vi "Intake_Execute.vi"() -> ()   [LabVIEW 2019]
uses:
  <vilib>/Rock Robotics/WPI/Solenoid/WPI_SolenoidValue.ctl
  Globals/Intake_Globals.vi
  <vilib>/Rock Robotics/WPI/ThirdParty/REV Robotics/SPARK MAX/Typedef/Spark MAX Control Type.ctl
panel:
  in  "Intake_Speed":dbl
  out "Intake_Extend":T1=enum."Reverse"
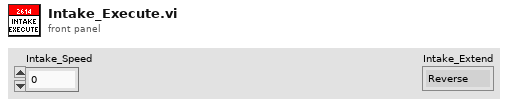
[diagram p1: front panel]
types:
  T1 = typedef "WPI_SolenoidValue.ctl" = enum16{"Off", "On", "Forward", "Reverse"}
  T2 = typedef "WPI_MotorControlDeviceRef.ctl" = cluster{"DeviceStatus":errorcluster, "Type":T3, "PWM":cluster{"PWM Channel":T4, "DeadBand":T5}, "CAN":cluster{"Device Number":u8, "SetOutput VI Ref":variant, "GetOutput VI Ref":variant, "Enable VI Ref":variant, "Disable VI Ref":variant, "Data":variant}, "Invert":bool, "DIO PWM":cluster{"PWM \"Enable\" Channel":T4, "DIOChannel":T6, "PWM Rate":dbl}}
  T3 = typedef "WPI_MotorControlType.ctl" = enum16{"PWM", "CAN", "DIO PWM"}
  T4 = typedef "FPGA_DIOPWMChannel.ctl" = enum8{"PWM 0", "PWM 1", "PWM 2", "PWM 3", "PWM 4", "PWM 5", "PWM 6", "PWM 7", "PWM 8", "PWM 9", "PWM MXP 0", "PWM MXP 1", "PWM MXP 2", "PWM MXP 3", "PWM MXP 4", "PWM MXP 5", "PWM MXP 6", "PWM MXP 7", "PWM MXP 8", "PWM MXP 9", "Invalid"}
  T5 = typedef "WPI_PWMDeadband.ctl" = cluster{"Name":string, "maxPositivePwm":i32, "minPositivePwm":i32, "centerPwm":i32, "maxNegativePwm":i32, "minNegativePwm":i32, "angularRange":u16}
  T6 = typedef "FPGA_DIOChannel.ctl" = enum8{"DIO 0", "DIO 1", "DIO 2", "DIO 3", "DIO 4", "DIO 5", "DIO 6", "DIO 7", "DIO 8", "DIO 9", "DIO MXP 0", "DIO MXP 1", "DIO MXP 2", "DIO MXP 3", "DIO MXP 4", "DIO MXP 5", "DIO MXP 6", "DIO MXP 7", "DIO MXP 8", "DIO MXP 9", "DIO MXP 10", "DIO MXP 11", "DIO MXP 12", "DIO MXP 13", "DIO MXP 14", "DIO MXP 15", "SPI Port CS1", "SPI Port CS2", "SPI Port CS3", "SPI Port MISO", "SPI Port MOSI", "Invalid"}
  T7 = typedef "Spark MAX Control Type.ctl" = enum16{"Percent VBus", "Voltage", "Velocity", "Position", "Smart Motion", "Current", "Smart Velocity"}
  T8 = typedef "Intake_Cluster.ctl" = cluster{"Control_State":T9, "Intake_On":bool, "Intake_Extended":bool, "Intake_Throttle":dbl}
  T9 = typedef "Intake_States.ctl" = enum16{"Manual_Control"}
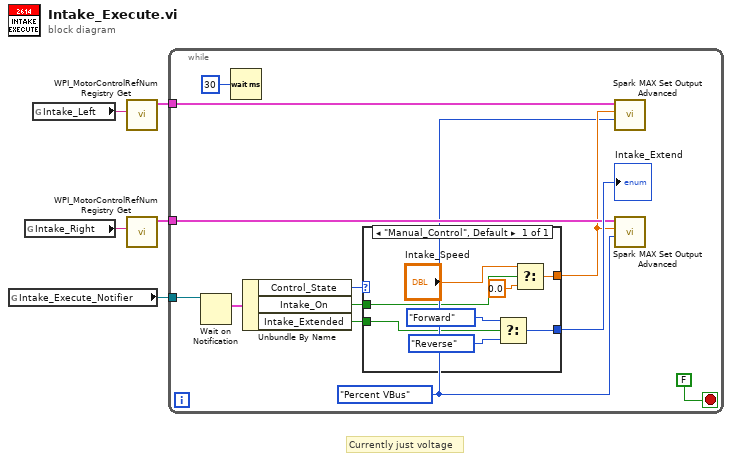
[diagram p0: block diagram]
diagram:
  # "Currently just voltage"
  n1 = global read "Intake_Globals.vi" "Intake_Execute_Notifier"() -> (w5:refnum<notifier>)
  n2 = global read "Intake_Globals.vi" "Intake_Right"() -> (w4:string)
  n3 = global read "Intake_Globals.vi" "Intake_Left"() -> (w3:string)
  n4 = call <vilib>:"WPI_MotorControlRefNum Registry Get.vi"("refnum name"=w3) -> ("MotorControlDevRef"=w2:T2)  [unwired: 9 in, 1 out]
  n5 = call <vilib>:"WPI_MotorControlRefNum Registry Get.vi"("refnum name"=w4) -> ("MotorControlDevRef"=w1:T2)  [unwired: 9 in, 1 out]
  n6 = while {
    tunnel: w5 -> [w16]
    tunnel: w2 -> [w9]
    tunnel: w1 -> [w8]
    stop <- FALSE stop-if-true
    w6 = Spark_MAX_Control_Type."Percent VBus" ("Control Mode")
    n7 = Wait on Notification(notifier=w16) -> (notification=w15:T8)  [unwired: 3 in, 3 out]
    n8 = Wait (ms)(milliseconds to wait=u32 30) -> ()  [unwired: 1 out]
    n9 = Unbundle By Name(w15) -> ("Control_State"=w14:T9, "Intake_On"=w11:bool, "Intake_Extended"=w13:bool)
    n10 = case shown="\"Manual_Control\", Default" w14 {
      tunnel: w13 -> [w24]
      tunnel: [w22] -> w12
      tunnel: w11 -> [w21]
      tunnel: [w18] -> w7
      frame "Manual_Control", Default {
        n11 = Select(t=WPI_SolenoidValue."Forward" ("Value"), s=w24, f=WPI_SolenoidValue."Reverse" ("Value")) -> (s? t:f=w22:T1)
        n12 = Select(t="Intake_Speed", s=w21, f=0.0) -> (s? t:f=w18:dbl)
      }
    }
    "Intake_Extend" <- w12
    n13 = call <vilib>:"Spark MAX Set Output Advanced.vi"("Control Mode"=w6, "Setpoint"=w7, "MotorControlDevRef"=w9) -> ()  [unwired: 7 in, 2 out]
    n14 = call <vilib>:"Spark MAX Set Output Advanced.vi"("Control Mode"=w6, "Setpoint"=w7, "MotorControlDevRef"=w8) -> ()  [unwired: 7 in, 2 out]
  }
